vi "Main.vi"() -> ()   [LabVIEW 2015]
uses:
  type defs/action buttons.ctl
  type defs/mode buttons.ctl
  type defs/state.ctl
  type defs/data.ctl
  <vilib>/vision/Image Controls.llb/IMAQ Image.ctl
  type defs/task.ctl
  <vilib>/myRIO/Instrument Drivers/Onboard IO/DIO/typedefs/DIO Reference.ctl
  <vilib>/myRIO/Common/Instrument Driver Framework/Utilities/typedefs/myRIO Generic Hardware Reference.ctl
  <vilib>/myRIO/Common/Instrument Driver Framework/Utilities/typedefs/Hardware Version Enum.ctl
  <vilib>/myRIO/Common/Instrument Driver Framework/Utilities/typedefs/myRIO v1.0 Reference.ctl
  <vilib>/myRIO/Common/Instrument Driver Framework/Utilities/typedefs/Generic FPGA Reference.ctl
  <vilib>/myRIO/Common/Instrument Driver Framework/myRIO v1.0/DIO/typedefs/DIO Channels List.ctl
  <vilib>/myRIO/Common/Instrument Driver Framework/myRIO v1.0/DIO/typedefs/DIO Channels Enum.ctl
  <vilib>/userdefined/High Color/nirio_resource_hc.ctl
  <vilib>/myRIO/Common/Instrument Driver Framework/Utilities/vis/Is FPGA Ref Available.vi
  <vilib>/myRIO/Common/Instrument Driver Framework/myRIO v1.0/DIO/vis/myRIO v1.1 Open DIO.vi
  <vilib>/myRIO/Instrument Drivers/Onboard IO/DIO/vis/Write.vi
  <vilib>/myRIO/Instrument Drivers/Onboard IO/DIO/vis/Read.vi
  <vilib>/myRIO/Common/Instrument Driver Framework/Utilities/vis/Validate Channels.vi
  <vilib>/myRIO/Common/Instrument Driver Framework/myRIO v1.0/DIO/vis/myRIO v1.0 Reserve DIO.vi
  <vilib>/myRIO/Common/Instrument Driver Framework/myRIO v1.0/Resource Manager/vis/myRIO v1.0 Reserve Channel List.vi
  <vilib>/myRIO/Common/Instrument Driver Framework/myRIO v1.0/DIO/vis/myRIO v1.0 Build MUX Configuration DIO.vi
  <vilib>/myRIO/Common/Instrument Driver Framework/myRIO v1.0/Resource Manager/vis/myRIO v1.0 Reserve Channel.vi
  <vilib>/myRIO/Common/Instrument Driver Framework/myRIO v1.0/Resource Manager/vis/myRIO v1.0 Unreserve Channel.vi
  <vilib>/myRIO/Common/Instrument Driver Framework/myRIO v1.0/Resource Manager/vis/myRIO v1.0 Create Configuration List.vi
  <vilib>/myRIO/Common/Instrument Driver Framework/myRIO v1.0/Resource Manager/vis/myRIO v1.0 Build Mutex Name.vi
  <vilib>/Utility/VariantDataType/GetNumericInfo.vi
  <vilib>/Utility/error.llb/Error Cluster From Error Code.vi
  <vilib>/myRIO/Common/Instrument Driver Framework/myRIO v1.0/myRIO v1.1 Open.vi
  <vilib>/myRIO/Common/Instrument Driver Framework/Utilities/vis/IO Manager.vi
  <vilib>/myRIO/Common/Instrument Driver Framework/Utilities/vis/Configuration Manager.vi
  <vilib>/myRIO/Common/Instrument Driver Framework/myRIO v1.0/Resource Manager/vis/myRIO v1.0 Configure IO.vi
  <vilib>/myRIO/Common/Instrument Driver Framework/myRIO v1.0/myRIO v1.0 Close.vi
  <vilib>/myRIO/Common/Instrument Driver Framework/myRIO v1.0/DIO/vis/myRIO v1.0 Write DIO.vi
  <vilib>/myRIO/Common/Instrument Driver Framework/myRIO v1.0/DIO/vis/myRIO v1.0 Read DIO.vi
  <vilib>/myRIO/Express VI/Onboard Devices/LED/LED Express VI.xnode
  <vilib>/myRIO/Instrument Drivers/Onboard IO/DIO/vis/myRIO DIO Open.xnode
  <vilib>/myRIO/Express VI/Onboard Devices/Button/Button Express VI.xnode
  <vilib>/vision/NI_Vision_Development_Module.lvlib
  <vilib>/myRIO/Instrument Drivers/Onboard IO/DIO/DIO.lvlib
panel:
  out "dTime States":T1[](array[typedef])
  out "dTime [ms]":u32[](array[numeric])
  in  "mode buttons":T2
  out "image display":T3(plugin-control)
  in  "action buttons":T4
  in  "Stop":bool
  # "FSM Optimized\nImage Rasterizer"
  # "This LabVIEW project attempts to optimize the Image Raster techniques used to obtain Laser Dot locations in the FOV in order to compare this algorithm against others."
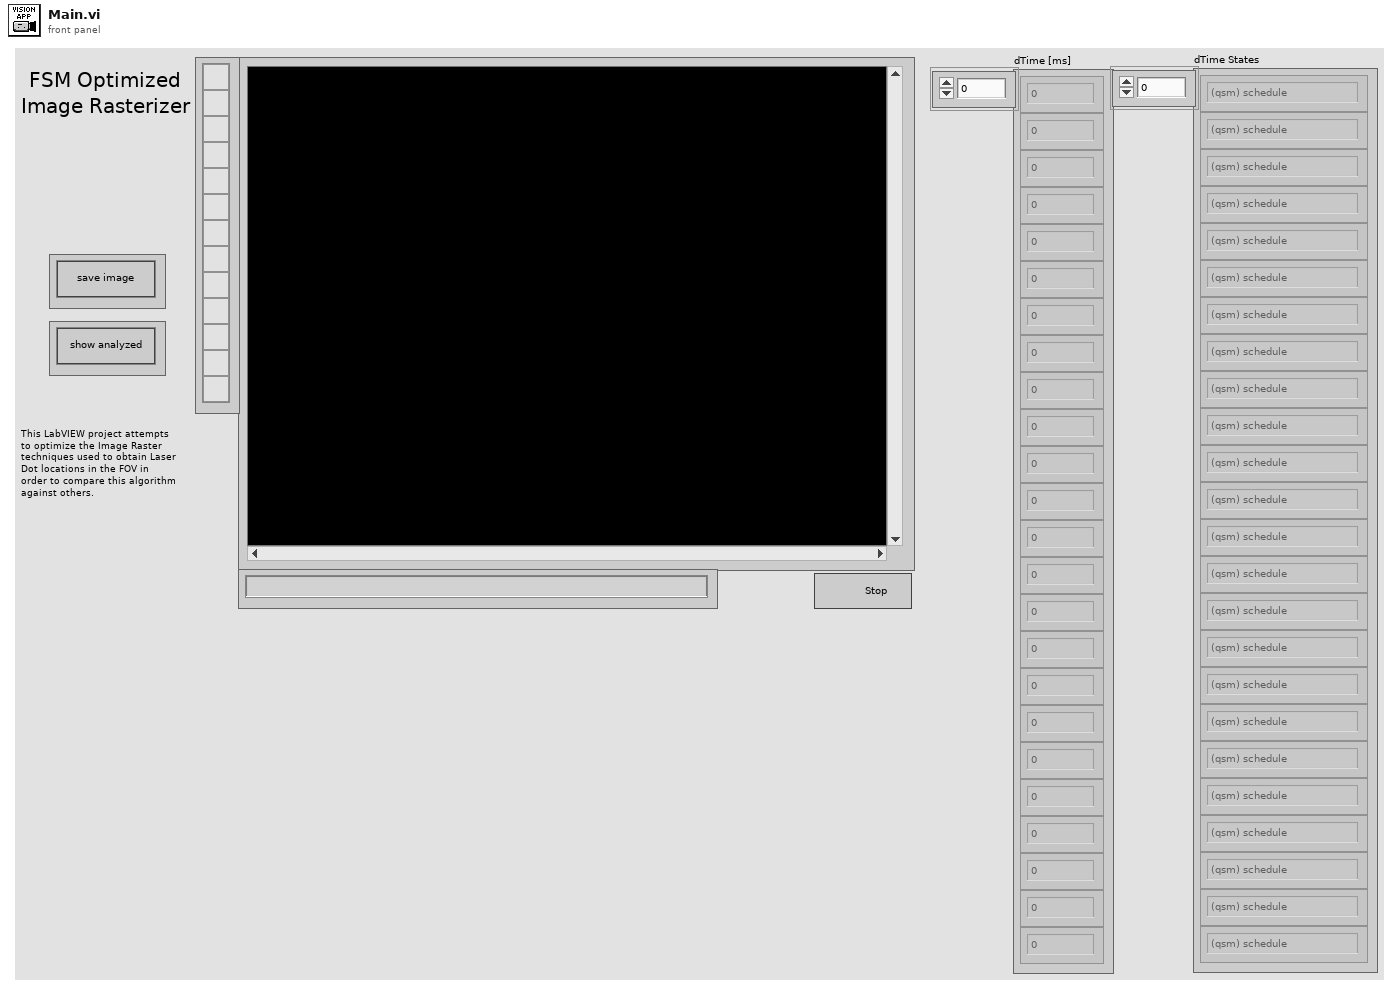
[diagram p1: front panel]
types:
  T1 = typedef "state.ctl" = enum16{"(qsm) schedule", "(qsm) initialize", "(qsm) release", "(qsm) clean up", "(qsm) shutdown", "(myRIO) initialize", "(myRIO) clean up", "(myRIO) update ports", "(image) get", "(image) analyze", "(image) overlay", "(image) show", "save image", "state A", "state B", "state C", "state D", "state E", "state F", "state G", "state H"}
  T2 = typedef "mode buttons.ctl" = cluster{"show analyzed":bool}
  T3 = typedef "IMAQ Image.ctl" = refnum<image>
  T4 = typedef "action buttons.ctl" = cluster{"save image":bool}
  T5 = typedef "DIO.lvlib/DIO Reference.ctl" = cluster{"myRIO Reference":T6, "DIO Channels List":T10}
  T6 = typedef "myRIO Generic Hardware Reference.ctl" = cluster{"myRIO Model":T7, "myRIO Hardware Reference":T8}
  T7 = typedef "Hardware Version Enum.ctl" = enum16{"Unknown", "myRIO-1900", "myRIO-1950", "roboRIO"}
  T8 = typedef "myRIO v1.0 Reference.ctl" = cluster{"Generic FPGA Reference":T9, "Allow multiple opens":bool}
  T9 = typedef "Generic FPGA Reference.ctl" = refnum<k20>
  T10 = typedef "DIO Channels List.ctl" = T11[]
  T11 = typedef "DIO Channels Enum.ctl" = enum16{"Not Connected", "C/DIO0", "C/DIO1", "C/DIO2", "C/DIO3", "C/DIO4", "C/DIO5", "C/DIO6", "C/DIO7", "A/DIO0", "A/DIO1", "A/DIO2", "A/DIO3", "A/DIO4", "A/DIO5", "A/DIO6", "A/DIO7", "A/DIO8", "A/DIO9", "A/DIO10", "A/DIO11", "A/DIO12", "A/DIO13", "A/DIO14", "A/DIO15", "B/DIO0", "B/DIO1", "B/DIO2", "B/DIO3", "B/DIO4", "B/DIO5", "B/DIO6", "B/DIO7", "B/DIO8", "B/DIO9", "B/DIO10", "B/DIO11", "B/DIO12", "B/DIO13", "B/DIO14", "B/DIO15", "LED0", "LED1", "LED2", "LED3", "Button0", "DIO/DIO0", "DIO/DIO1", "DIO/DIO2", "DIO/DIO3", "DIO/DIO4", "DIO/DIO5", "DIO/DIO6", "DIO/DIO7", "DIO/DIO8", "DIO/DIO9", "SPI/CS0", "SPI/CS1", "SPI/CS2", "SPI/CS3", "LED RADIO (Green)", "LED RADIO (Red)", "LED COMM (Green)", "LED COMM (Red)", "LED MODE (Green)", "LED MODE (Red)"}
  T12 = typedef "nirio_resource_hc.ctl" = tag
  T13 = typedef "data.ctl" = cluster{"save image":bool, "qsm":cluster{"Webcam image ref":T3, "Analyzed image ref":T3, "Stop webcam":bool}, "LaserDotLocation":cluster{"XLocation":i32, "YLocation":i32}}
  T14 = typedef "task.ctl" = T1[]
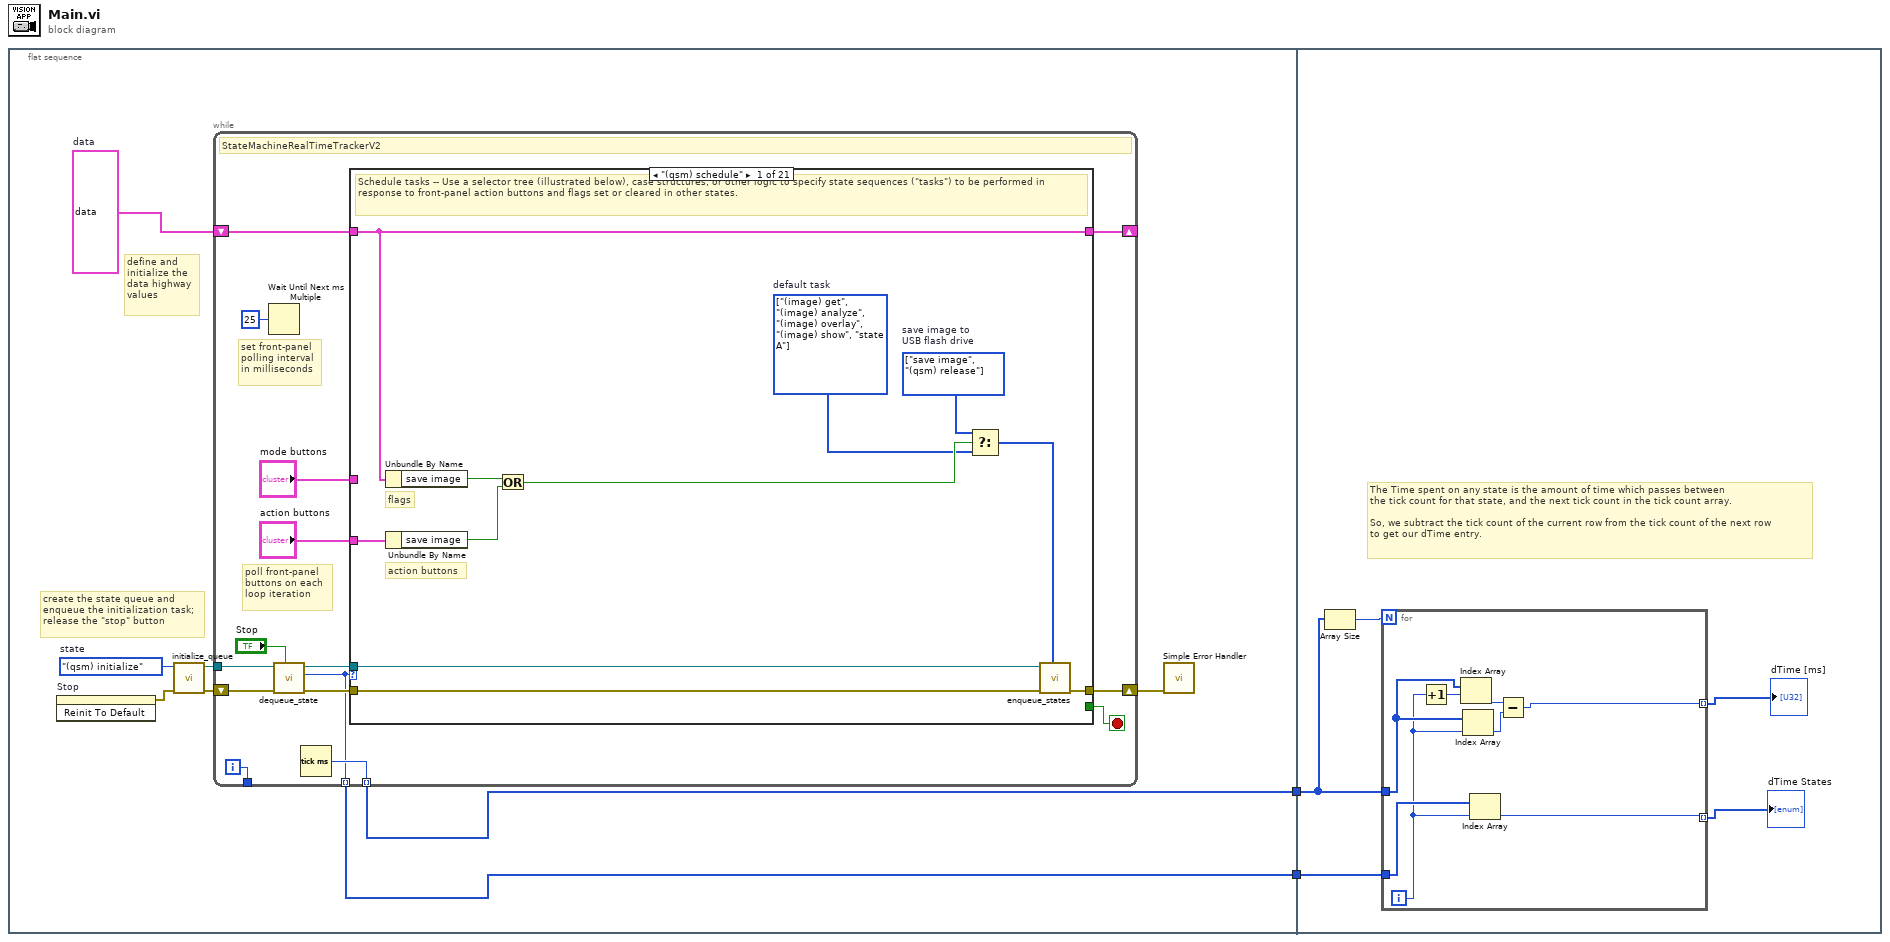
[diagram p0: block diagram]
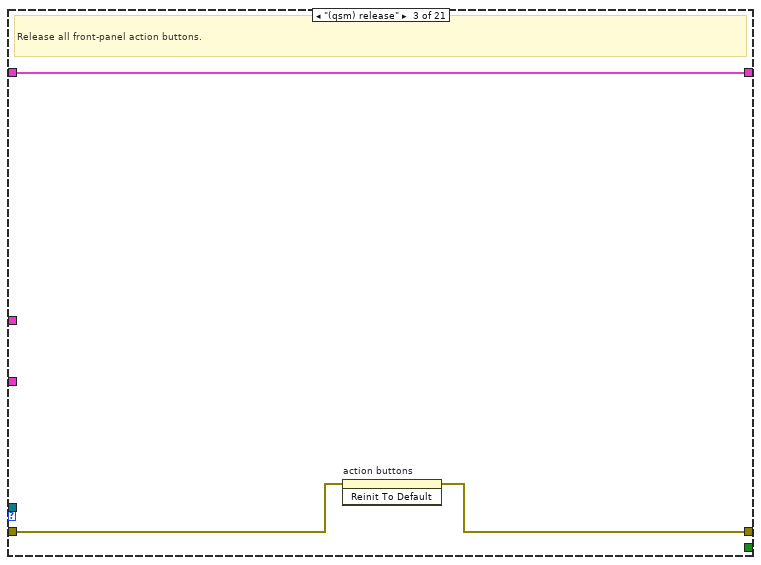
[diagram p3: hidden frame]
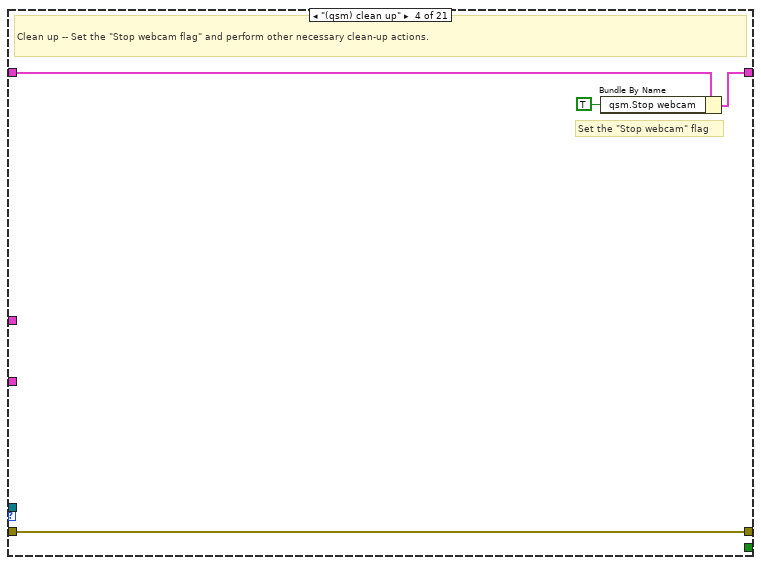
[diagram p4: hidden frame]
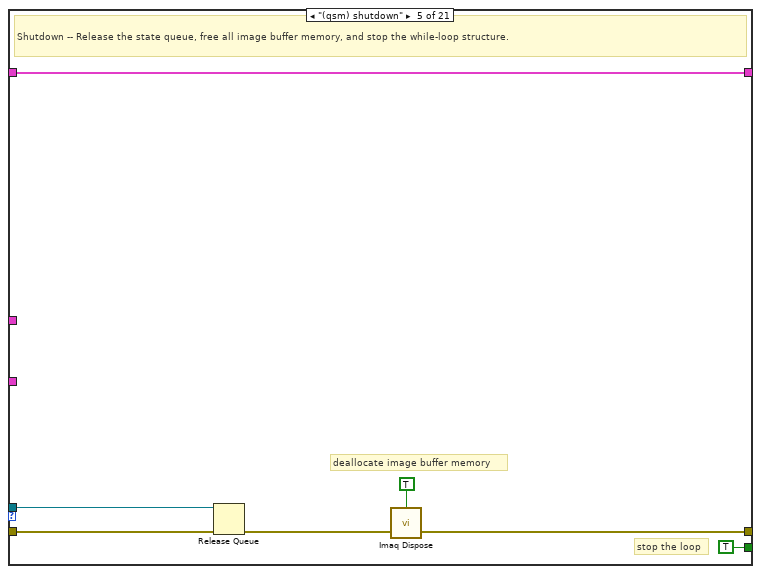
[diagram p5: hidden frame]
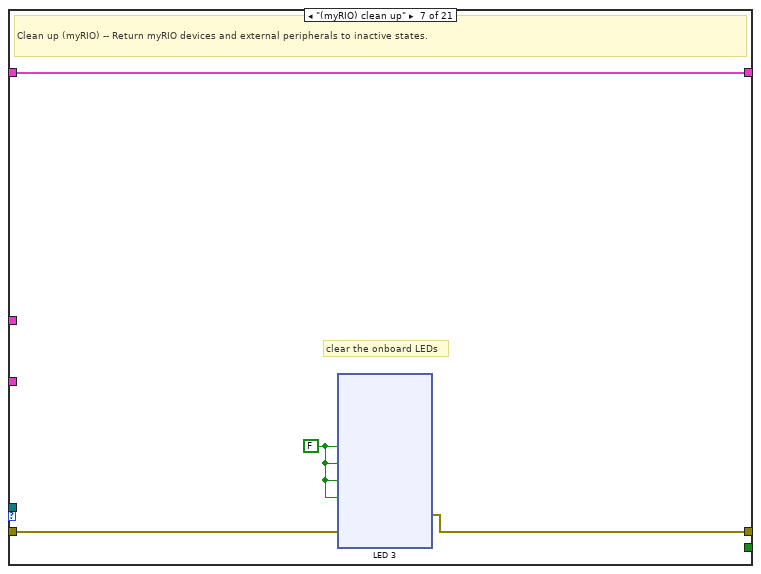
[diagram p7: hidden frame]
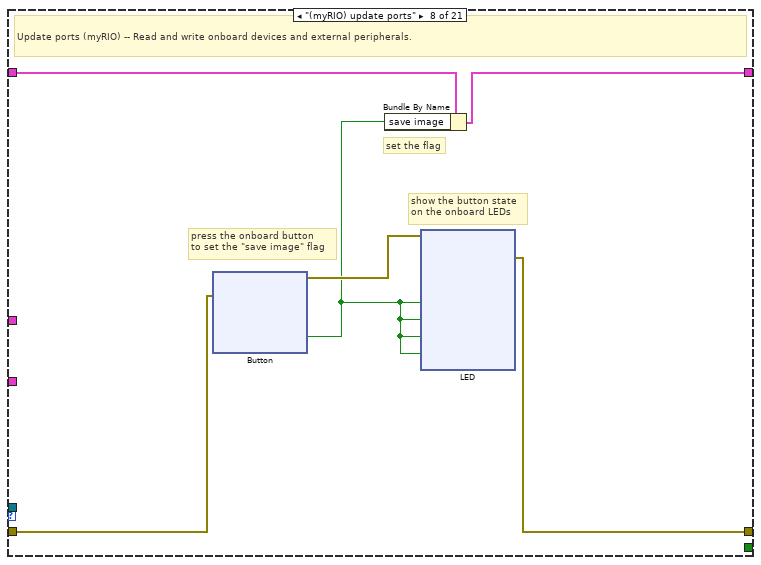
[diagram p8: hidden frame]
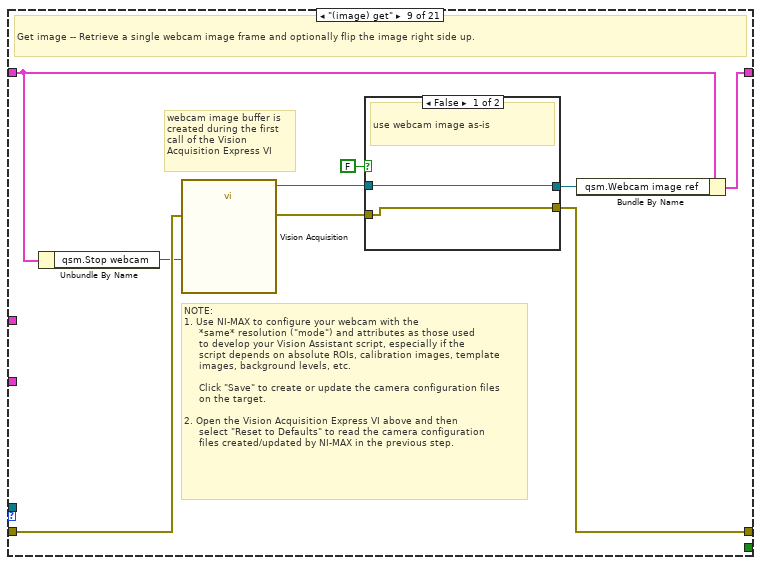
[diagram p9: hidden frame]
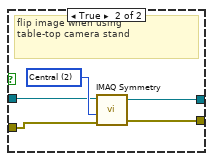
[diagram p10: hidden frame]
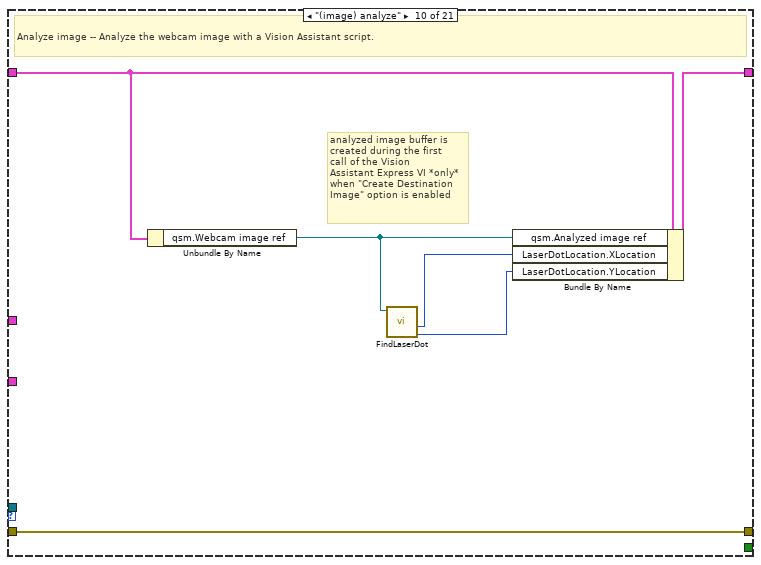
[diagram p11: hidden frame]
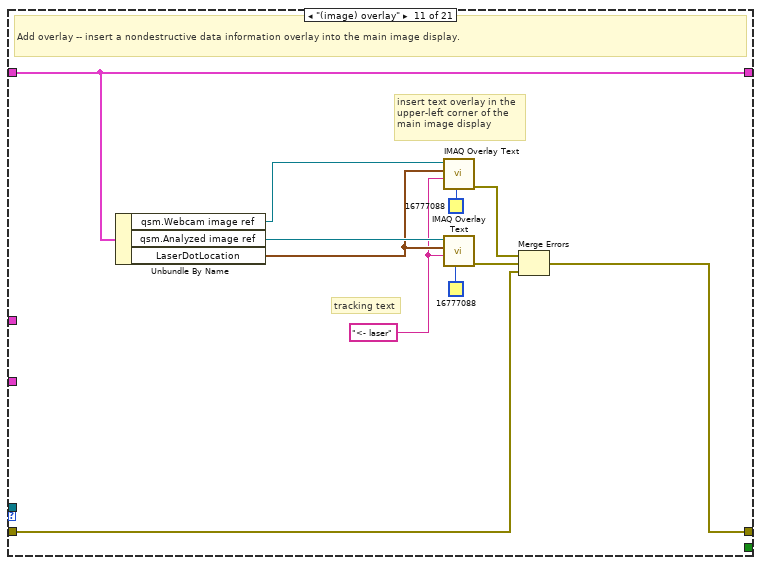
[diagram p12: hidden frame]
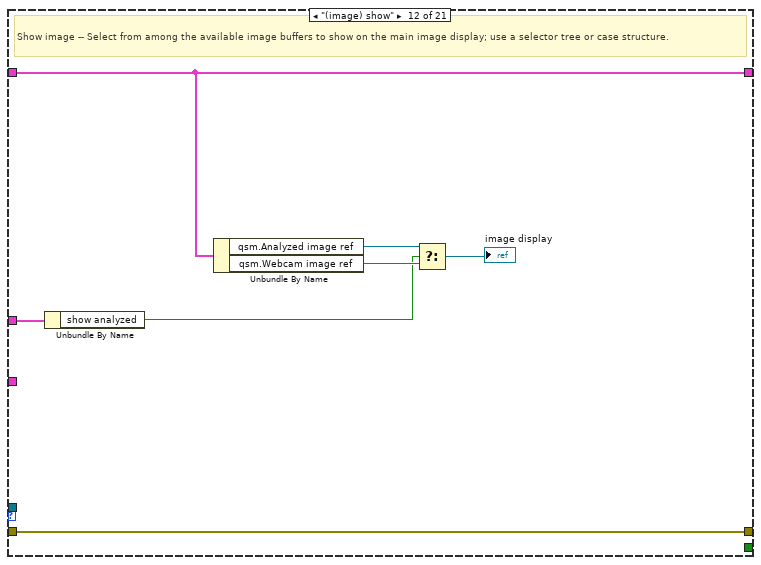
[diagram p13: hidden frame]
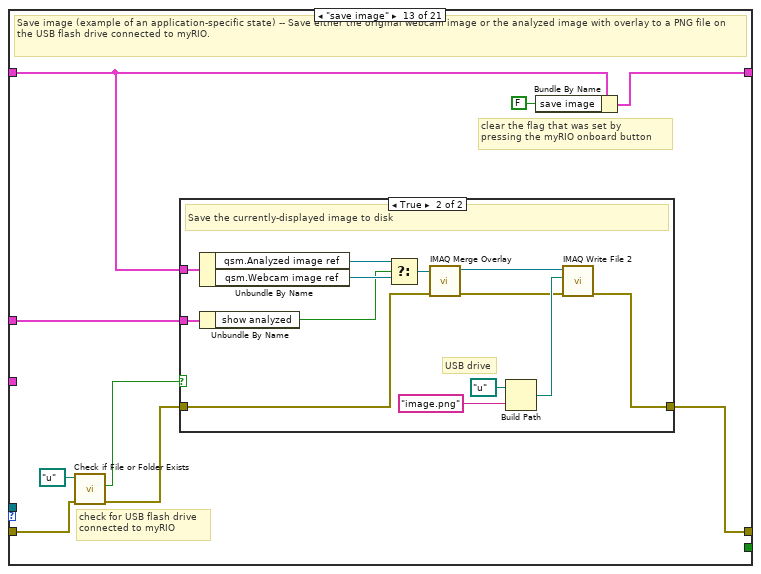
[diagram p14: hidden frame]
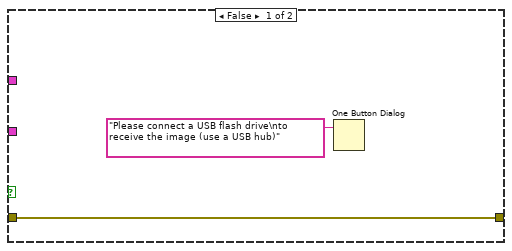
[diagram p15: hidden frame]
diagram:
  n1 = flat-sequence {
    tunnel: [w4] -> w2
    tunnel: [w3] -> w1
    tunnel: w2 -> [w258]
    tunnel: w1 -> [w260]
    frame #0 {
      w9 = T13 {"save image"=FALSE, "qsm"={"Webcam image ref"=refnum, "Analyzed image ref"=refnum, "Stop webcam"=FALSE}, "LaserDotLocation"={"XLocation"=0, "YLocation"=0}}  # data
      w5 = state."(qsm) initialize"  # state
      # "define and \ninitialize the \ndata highway\nvalues"
      # "create the state queue and\nenqueue the initialization task;\nrelease the \"stop\" button"
      n2 = invoke on="Stop" class="Bool" method="Reinit To Default"() -> (error out=w6:errorcluster)  [unwired: 3 in, 2 out]
      n3 = call "initialize_queue.vi"("error in (no error)"=w6, "state"=w5) -> ("error out"=w8:errorcluster, "queue out"=w7:refnum<queue>)  [unwired: 8 in]
      n4 = while {
        shift-right: [w25] -> w10
        shift-left: w8 -> [w18]
        tunnel: w7 -> [w19]
        shift-right: [w22] -> _
        shift-left: w9 -> [w23]
        tunnel: [w13] -> _
        tunnel: [w12] -> w4 mode=indexing
        tunnel: [w11] -> w3 mode=indexing
        i -> [w13]
        stop <- w21 stop-if-true
        # "set front-panel\npolling interval\nin milliseconds"
        # "poll front-panel\nbuttons on each\nloop iteration"
        # "StateMachineRealTimeTrackerV2"
        n5 = Wait Until Next ms Multiple(millisecond multiple=u32 25) -> ()  [unwired: 1 out]
        n6 = call "dequeue_state.vi"("stop"="Stop", "error in (no error)"=w18, "queue in"=w19) -> ("error out"=w20:errorcluster, "state"=w11:T1, "queue out"=w16:refnum<queue>)  [unwired: 6 in]
        n7 = Tick Count (ms)() -> (millisecond timer value=w12:u32)
        n8 = case shown="\"(qsm) schedule\"" w11 {
          tunnel: w20 -> [w32 w38 w40 w42 w51 w53 w56 w100 w184 w196 w199 w211 w220 w241 w243 w245 w247 w249 w250 w252 w255]
          tunnel: w16 -> [w33 _ _ _ w50 _ _ _ _ _ _ _ _ _ _ _ _ _ _ _ _]
          tunnel: [w34 w38 w39 w42 w46 w53 w55 w98 w179 w196 w203 w211 w218 w241 w243 w245 w247 w249 w250 w252 w255] -> w25
          tunnel: "action buttons" -> [w36 _ _ _ _ _ _ _ _ _ _ _ _ _ _ _ _ _ _ _ _]
          tunnel: w23 -> [w35 w37 w41 w44 w49 w54 w58 w102 w177 w195 w201 w212 w224 w240 w242 w244 w246 w248 w251 w253 w254]
          tunnel: [w35 w37 w41 w43 w49 w54 w58 w101 w183 w197 w201 w212 w223 w240 w242 w244 w246 w248 w251 w253 w254] -> w22
          tunnel: [_ _ _ _ TRUE _ _ _ _ _ _ _ _ _ _ _ _ _ _ _ _] -> w21
          tunnel: "mode buttons" -> [_ _ _ _ _ _ _ _ _ _ _ w210 w219 _ _ _ _ _ _ _ _]
          frame "(qsm) schedule" {
            w28 = T14 [enum."save image", enum."(qsm) release"] items=["(qsm) schedule", "(qsm) initialize", "(qsm) release", "(qsm) clean up", "(qsm) shutdown", "(myRIO) initialize", "(myRIO) clean up", "(myRIO) update ports", "(image) get", "(image) analyze", "(image) overlay", "(image) show", "save image", "state A", "state B", "state C", "state D", "state E", "state F", "state G", "state H"]  # save image to USB flash drive
            w26 = T14 [enum."(image) get", enum."(image) analyze", enum."(image) overlay", enum."(image) show", enum."state A"] items=["(qsm) schedule", "(qsm) initialize", "(qsm) release", "(qsm) clean up", "(qsm) shutdown", "(myRIO) initialize", "(myRIO) clean up", "(myRIO) update ports", "(image) get", "(image) analyze", "(image) overlay", "(image) show", "save image", "state A", "state B", "state C", "state D", "state E", "state F", "state G", "state H"]  # default task
            # "action buttons"
            # "flags"
            # "Schedule tasks -- Use a selector tree (illustrated below), case structures, or other logic to specify state sequences (\"tasks\") to be performed in response to front-panel action buttons and flags set or cleared in other states."
            n9 = Unbundle By Name "Unbundle By Name"(w35) -> ("save image"=w31:bool)
            n10 = Unbundle By Name(w36) -> ("save image"=w30:bool)
            n11 = Or(x=w31, y=w30) -> (x .or. y?=w29:bool)
            n12 = Select(t=w28, s=w29, f=w26) -> (s? t:f=w27:T14)
            n13 = call "enqueue_states.vi"("task"=w27, "error in"=w32, "queue in"=w33) -> ("error out"=w34:errorcluster)  [unwired: 7 in, 1 out]
          }
          frame "(qsm) initialize" {
            # "Initialize -- Allocate memory for additional image buffers, if necessary, and perform other one-time initialization steps."
          }
          frame "(qsm) release" {
            # "Release all front-panel action buttons."
            n14 = invoke on="action buttons" class="Clust (strict)" method="Reinit To Default"(error in=w40) -> (error out=w39:errorcluster)  [unwired: 2 in, 2 out]
          }
          frame "(qsm) clean up" {
            # "Set the \"Stop webcam\" flag"
            # "Clean up -- Set the \"Stop webcam flag\" and perform other necessary clean-up actions."
            n15 = Bundle By Name(cluster=w44, "qsm.Stop webcam"=TRUE) -> (w43:T13)
          }
          frame "(qsm) shutdown" {
            # "deallocate image buffer memory"
            # "stop the loop"
            # "Shutdown -- Release the state queue, free all image buffer memory, and stop the while-loop structure."
            n16 = Release Queue(queue=w50, error in (no error)=w51) -> (error out=w47:errorcluster)  [unwired: 1 in, 2 out]
            n17 = call "Imaq Dispose"("All Images? (No)"=TRUE, "error in (no error)"=w47) -> ("error out"=w46:errorcluster)  [unwired: 4 in]
          }
          frame "(myRIO) initialize" {
            # "Initialize (myRIO) -- Open channels, configure devices, send setup strings to peripherals, etc."
          }
          frame "(myRIO) clean up" {
            w57 = FALSE ("LED3")
            # "clear the onboard LEDs"
            # "Clean up (myRIO) -- Return myRIO devices and external peripherals to inactive states."
            n18 = xnode "LED 3"("LED0"=w57, "LED1"=w57, "LED2"=w57, "LED3"=w57, "error in (no error)"=w56) -> ("error out"=w55:errorcluster)
          }
          frame "(myRIO) update ports" {
            # "show the button state\non the onboard LEDs"
            # "set the flag"
            # "press the onboard button\nto set the \"save image\" flag"
            # "Update ports (myRIO) -- Read and write onboard devices and external peripherals."
            n19 = xnode "Button"("error in (no error)"=w100) -> ("Value"=w97:bool, "error out"=w99:errorcluster)
            n20 = Bundle By Name "Bundle By Name"(cluster=w102, "save image"=w97) -> (w101:T13)
            n21 = xnode "LED"("LED0"=w97, "LED1"=w97, "LED2"=w97, "LED3"=w97, "error in (no error)"=w99) -> ("error out"=w98:errorcluster)
          }
          frame "(image) get" {
            # "webcam image buffer is\ncreated during the first\ncall of the Vision\nAcquisition Express VI"
            # "NOTE:\n1. Use NI-MAX to configure your webcam with the\n     *same* resolution (\"mode\") and attributes as those used \n     to develop your Vision Assistant script, especially if the\n     script depends on absolute ROIs, calibration images, template\n     images, background levels, etc.\n \n     Click \"Save\" to create or update the camera configuration files\n     on the target.\n\n2. Open the Vision Acquisition Express VI above and then\n     select \"Reset to Defaults\" to read the camera configuration\n     files created/updated by NI-MAX in the previous step."
            # "Get image -- Retrieve a single webcam image frame and optionally flip the image right side up."
            n22 = Unbundle By Name(w177) -> ("qsm.Stop webcam"=w176:bool)
            n23 = call "Vision Acquisition"("Stop (F)"=w176, "error in"=w184) -> ("Image Out"=w182:T3, "error out"=w180:errorcluster)  [unwired: 23 in, 1 out]
            n24 = case shown="False" FALSE {
              tunnel: w182 -> [w186 w190]
              tunnel: [w186 w189] -> w181
              tunnel: w180 -> [w185 w188]
              tunnel: [w185 w187] -> w179
              frame False {
                # "use webcam image as-is"
              }
              frame True {
                w191 = u32 2 items=["Horizontal", "Vertical", "Central", "1st Diagonal", "2nd Diagonal"] ("Type of Symmetry")
                # "flip image when using\ntable-top camera stand"
                n25 = call "IMAQ Symmetry"("error in (no error)"=w188, "Type of Symmetry"=w191, "Image Src"=w190) -> ("error out"=w187:errorcluster, "Image Dst Out"=w189:T3)  [unwired: 2 in]
              }
            }
            n26 = Bundle By Name(cluster=w177, "qsm.Webcam image ref"=w181) -> (w183:T13)
          }
          frame "(image) analyze" {
            # "analyzed image buffer is\ncreated during the first\ncall of the Vision\nAssistant Express VI *only*\nwhen \"Create Destination\nImage\" option is enabled"
            # "Analyze image -- Analyze the webcam image with a Vision Assistant script."
            n27 = Unbundle By Name "Unbundle By Name"(w195) -> ("qsm.Webcam image ref"=w194:T3)
            n28 = call "FindLaserDot.vi"("Image Input"=w194) -> ("Y Location"=w192:i32, "X Location"=w193:i32)  [unwired: 7 in, 2 out]
            n29 = Bundle By Name "Bundle By Name"(cluster=w195, "qsm.Analyzed image ref"=w194, "LaserDotLocation.XLocation"=w193, "LaserDotLocation.YLocation"=w192) -> (w197:T13)
          }
          frame "(image) overlay" {
            w198 = "<- laser" ("format string")
            # "tracking text"
            # "insert text overlay in the\nupper-left corner of the \nmain image display"
            # "Add overlay -- insert a nondestructive data information overlay into the main image display."
            n30 = Unbundle By Name "Unbundle By Name"(w201) -> ("qsm.Webcam image ref"=w205:T3, "qsm.Analyzed image ref"=w208:T3, "LaserDotLocation"=w200:cluster{"XLocation":i32, "YLocation":i32})
            n31 = call "IMAQ Overlay Text"("Text Color (black)"=u32 16777088, "String"=w198, "Origin"=w200, "Image"=w205) -> ("error out"=w202:errorcluster)  [unwired: 6 in, 1 out]
            n32 = call "IMAQ Overlay Text"("Text Color (black)"=u32 16777088, "String"=w198, "Origin"=w200, "Image"=w208) -> ("error out"=w204:errorcluster)  [unwired: 6 in, 1 out]
            n33 = Merge Errors "Merge Errors"(w202, w204, w199) -> (w203:errorcluster)
          }
          frame "(image) show" {
            # "Show image -- Select from among the available image buffers to show on the main image display; use a selector tree or case structure."
            n34 = Unbundle By Name "Unbundle By Name"(w210) -> ("show analyzed"=w209:bool)
            n35 = Unbundle By Name "Unbundle By Name"(w212) -> ("qsm.Analyzed image ref"=w215:T3, "qsm.Webcam image ref"=w214:T3)
            n36 = Select(t=w215, s=w209, f=w214) -> (s? t:f=→"image display":T3)
          }
          frame "save image" {
            # "check for USB flash drive\nconnected to myRIO"
            # "clear the flag that was set by\npressing the myRIO onboard button"
            # "Save image (example of an application-specific state) -- Save either the original webcam image or the analyzed image with overlay to a PNG file on the USB flash drive connected to myRIO."
            n37 = call <vilib>:"Check if File or Folder Exists.vi"("error in (no error)"=w220, "path"=path "u:/") -> ("error out"=w216:errorcluster, "file or folder exists?"=w217:bool)  [unwired: 7 in, 1 out]
            n38 = case shown="True" w217 {
              tunnel: w224 -> [_ w235]
              tunnel: w219 -> [_ w234]
              tunnel: [w225 w232] -> w218
              tunnel: w216 -> [w225 w230]
              frame False {
                n39 = One Button Dialog(message="Please connect a USB flash drive\nto receive the image (use a USB hub)") -> ()  [unwired: 1 in, 1 out]
              }
              frame True {
                # "USB drive"
                # "Save the currently-displayed image to disk"
                n40 = Unbundle By Name(w235) -> ("qsm.Analyzed image ref"=w229:T3, "qsm.Webcam image ref"=w236:T3)
                n41 = Unbundle By Name(w234) -> ("show analyzed"=w231:bool)
                n42 = Select(t=w229, s=w231, f=w236) -> (s? t:f=w228:T3)
                n43 = call "IMAQ Merge Overlay"("error in (no error)"=w230, "Image Src"=w228) -> ("error out"=w237:errorcluster, "Image Dst Out"=w227:T3)  [unwired: 8 in]
                n44 = Build Path(base path=path "u:/", name or relative path="image.png") -> (appended path=w238:path)
                n45 = call-poly "IMAQ Write File 2"("error in (no error)"=w237, "File Path"=w238, "Image"=w227) -> ("error out"=w232:errorcluster)  [unwired: 7 in, 1 out]
              }
            }
            n46 = Bundle By Name(cluster=w224, "save image"=FALSE) -> (w223:T13)
          }
          frame "state A" {
            # "Expansion State A"
          }
          frame "state B" {
            # "Expansion State B"
          }
          frame "state C" {
            # "Expansion State C"
          }
          frame "state D" {
            # "Expansion State D"
          }
          frame "state E" {
            # "Expansion State E"
          }
          frame "state F" {
            # "Expansion State F"
          }
          frame "state G" {
            # "Expansion State G"
          }
          frame "state H" {
            # "Expansion State H"
          }
        }
      }
      n47 = call <vilib>:"Simple Error Handler.vi"("error in (no error)"=w10) -> ()  [unwired: 4 in, 5 out]
    }
    frame #1 {
      # "The Time spent on any state is the amount of time which passes between\nthe tick count for that state, and the next tick count in the tick count array.  \n\nSo, we subtract the tick count of the current row from the tick count of the next row\nto get our dTime entry."
      n48 = Array Size(array=w258) -> (size(s)=w259:i32)
      n49 = for {
        N: w259 -> [_]
        tunnel: w258 -> [w266]
        tunnel: w260 -> [w268]
        tunnel: [w263] -> w256 mode=indexing
        tunnel: [w262] -> w257 mode=indexing
        i -> [w261]
        n50 = Increment(x=w261) -> (x+1=w267:i32)
        n51 = Index Array(array=w266, index=w267) -> (element=w265:u32)
        n52 = Index Array(array=w266, index=w261) -> (element=w264:u32)
        n53 = Index Array(array=w268, index=w261) -> (element=w262:T1)
        n54 = Subtract(x=w265, y=w264) -> (x-y=w263:u32)
      }
      "dTime [ms]" <- w256
      "dTime States" <- w257
    }
  }
